vi "Split bytes.vi"(8 "error in":errorcluster, 9 "count (1)":i32=1, 10 "start index (0)":i32, 11 "bytes in":u8[](array[numeric])) -> (0 "error out":errorcluster, 2 "selected bytes":u8[](array[numeric]), 3 "remaining bytes":u8[](array[numeric]), 4 "before bytes":u8[](array[numeric]))   [LabVIEW 2020, in "MessagePack.lvlib"]
uses:
  MessagePack.lvlib
  <vilib>/ErrorRing/Error Ring.xnode
  <vilib>/Utility/error.llb/Error Cluster From Error Code.vi
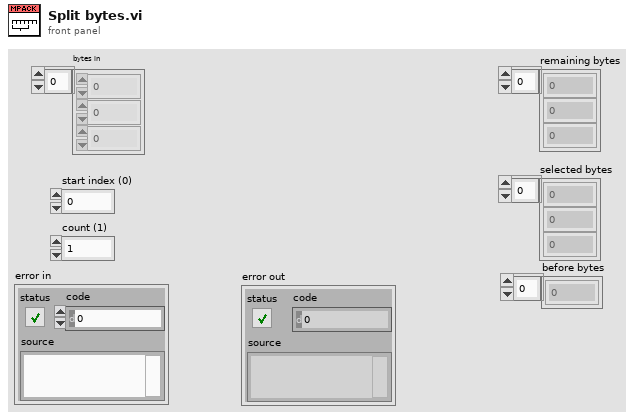
[diagram p1: front panel]
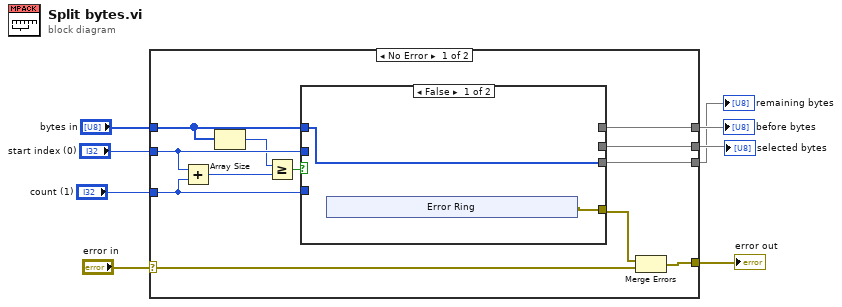
[diagram p0: block diagram]
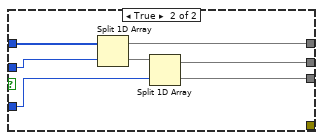
[diagram p2: hidden frame]
diagram:
  n1 = case shown="No Error" "error in" {
    selector: "error in" -> [w19 w35]
    tunnel: [w17 w35] -> w7
    tunnel: "start index (0)" -> [w13 _]
    tunnel: "bytes in" -> [w11 w34]
    tunnel: "count (1)" -> [w12 _]
    tunnel: [w16 _] -> w3
    tunnel: [w15 _] -> w2
    tunnel: [w14 w34] -> w1
    frame No Error {
      n2 = Add(x=w13, y=w12) -> (x+y=w9:i32)
      n3 = Array Size(array=w11) -> (size(s)=w10:i32)
      n4 = Greater Or Equal?(x=w10, y=w9) -> (x >= y?=w20:bool)
      n5 = case shown="False" w20 {
        tunnel: [w22 _] -> w18
        tunnel: w11 -> [w21 w33]
        tunnel: w13 -> [_ w30]
        tunnel: [_ w32] -> w16
        tunnel: w12 -> [_ w27]
        tunnel: [_ w29] -> w15
        tunnel: [w21 w28] -> w14
        frame False {
          n6 = xnode "Error Ring"() -> ("error out"=w22:errorcluster)
        }
        frame True {
          n7 = Split 1D Array(array=w33, index=w30) -> (first subarray=w32:u8[], second subarray=w31:u8[])
          n8 = Split 1D Array(array=w31, index=w27) -> (first subarray=w29:u8[], second subarray=w28:u8[])
        }
      }
      n9 = Merge Errors(w18, w19) -> (w17:errorcluster)
    }
    frame Error {
    }
  }
  "error out" <- w7
  "selected bytes" <- w2
  "remaining bytes" <- w1
  "before bytes" <- w3
